vi "Load Modes.vi"(2 "Poke Path":string[](array[string]), 3 "Practical Mode Path":string[](array[string]), 4 "Theoretical Mode Path":string[](array[string]), 5 "Base File Path":path) -> ()   [LabVIEW 2014]
uses:
  Controls/Standard Action.ctl
  <vilib>/Utility/file.llb/Read From Spreadsheet File (DBL).vi
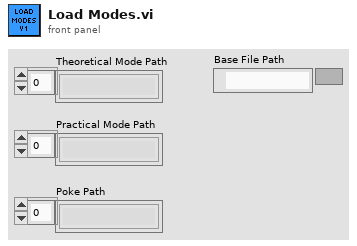
[diagram p1: front panel]
types:
  T1 = typedef "Standard Action.ctl" = enum16{"Read", "Write"}
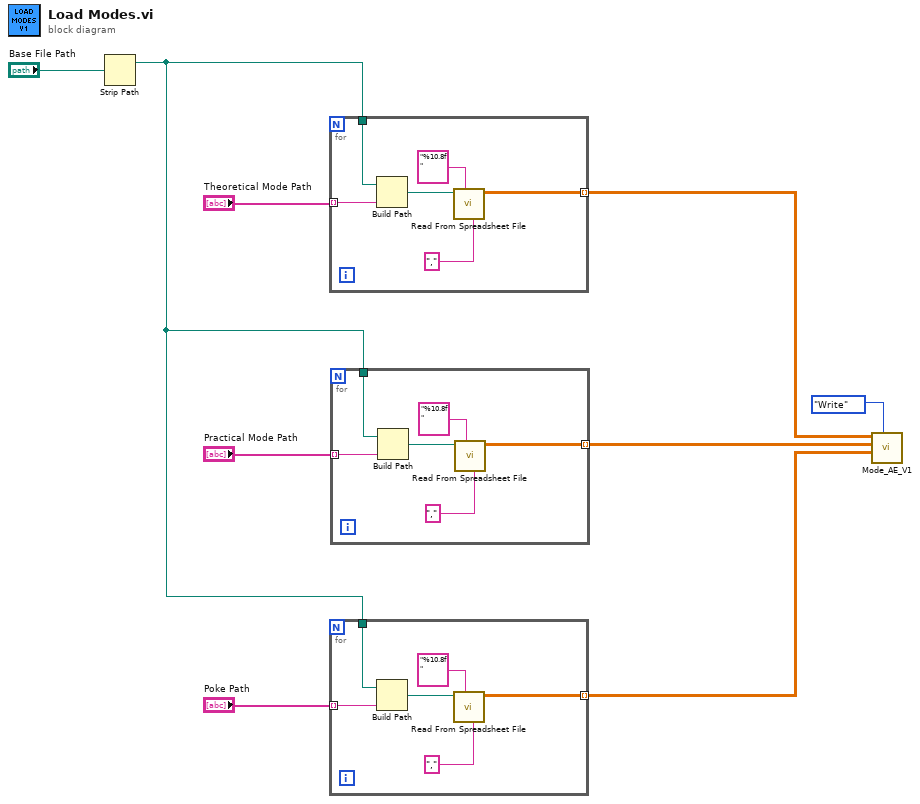
[diagram p0: block diagram]
diagram:
  n1 = Strip Path(path="Base File Path") -> (stripped path=w5:path)  [unwired: 1 out]
  n2 = for {
    tunnel: w5 -> [w13]
    tunnel: "Theoretical Mode Path" -> [w11] mode=indexing
    tunnel: [w10] -> w3 mode=indexing
    n3 = Build Path(base path=w13, name or relative path=w11) -> (appended path=w14:path)
    n4 = call-poly <vilib>:"Read From Spreadsheet File.vi"("delimiter (\\t)"="," ("delimiter (\\t)"), "format (%.3f)"="%10.8f", "file path (dialog if empty)"=w14) -> ("all rows"=w10:dbl[][])  [unwired: 2 in, 6 out]
  }
  n5 = for {
    tunnel: w5 -> [w19]
    tunnel: "Poke Path" -> [w17] mode=indexing
    tunnel: [w16] -> w1 mode=indexing
    n6 = Build Path(base path=w19, name or relative path=w17) -> (appended path=w20:path)
    n7 = call-poly <vilib>:"Read From Spreadsheet File.vi"("delimiter (\\t)"="," ("delimiter (\\t)"), "format (%.3f)"="%10.8f", "file path (dialog if empty)"=w20) -> ("all rows"=w16:dbl[][])  [unwired: 2 in, 6 out]
  }
  n8 = for {
    tunnel: w5 -> [w25]
    tunnel: "Practical Mode Path" -> [w23] mode=indexing
    tunnel: [w22] -> w2 mode=indexing
    n9 = Build Path(base path=w25, name or relative path=w23) -> (appended path=w26:path)
    n10 = call-poly <vilib>:"Read From Spreadsheet File.vi"("delimiter (\\t)"="," ("delimiter (\\t)"), "format (%.3f)"="%10.8f", "file path (dialog if empty)"=w26) -> ("all rows"=w22:dbl[][])  [unwired: 2 in, 6 out]
  }
  n11 = call "Mode_AE_V1.vi"("Action"=Standard_Action."Write", "Poke Mode In"=w1, "Practical Mode In"=w2, "Theoretical Mode In"=w3) -> ()  [unwired: 4 in, 3 out]
